vi "Draw Overlay.vi"(0 "Image (in)":T1, 1 "Image Width (in)":i32, 2 "Image Height (in)":i32, 3 "X Center (in)":sgl[](array[numeric]), 4 "Y Center (in)":sgl[](array[numeric]), 5 "Height (in)":sgl[](array[numeric]), 6 "Colors (in)":u32[](array[numeric]), 7 "Width (in)":sgl[](array[numeric]), 9 "Classes (in)":i32[](array[numeric])) -> (14 "Image (out)":T1)   [LabVIEW 2016]
uses:
  <vilib>/vision/Image Controls.llb/IMAQ Image.ctl
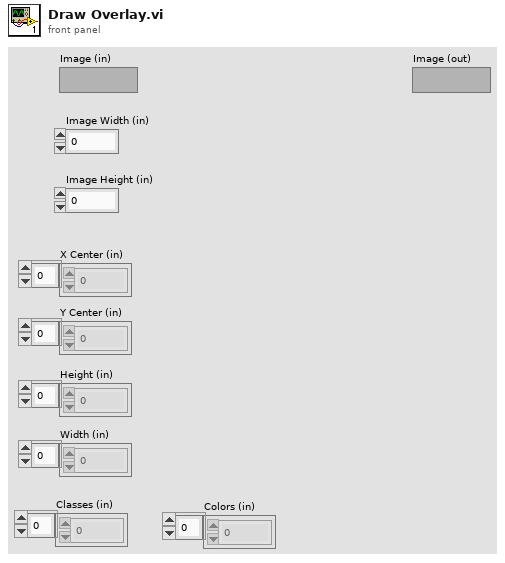
[diagram p1: front panel]
types:
  T1 = typedef "IMAQ Image.ctl" = refnum<image>
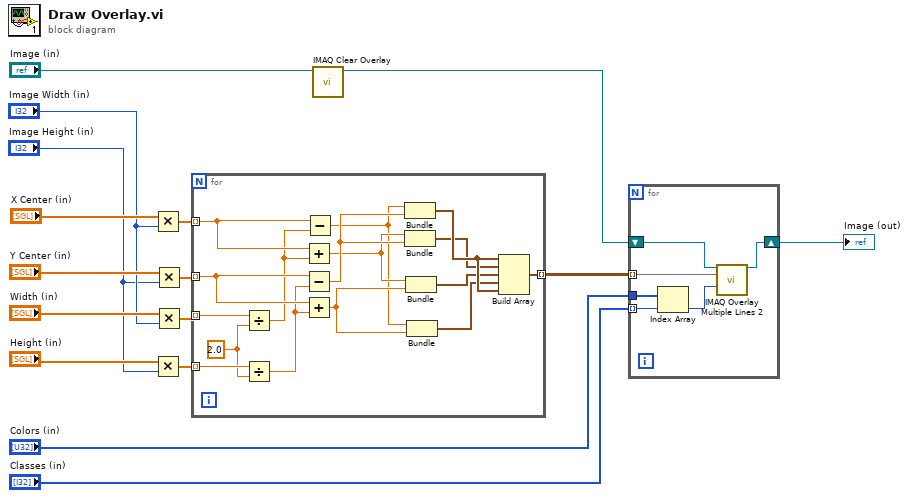
[diagram p0: block diagram]
diagram:
  n1 = Multiply(x="X Center (in)", y="Image Width (in)") -> (x*y=w4:sgl[])
  n2 = Multiply(x="Height (in)", y="Image Height (in)") -> (x*y=w7:sgl[])
  n3 = Multiply(x="Y Center (in)", y="Image Height (in)") -> (x*y=w5:sgl[])
  n4 = Multiply(x="Width (in)", y="Image Width (in)") -> (x*y=w6:sgl[])
  n5 = for {
    tunnel: w4 -> [w25] mode=indexing
    tunnel: w5 -> [w24] mode=indexing
    tunnel: w6 -> [w28] mode=indexing
    tunnel: w7 -> [w27] mode=indexing
    tunnel: [w17] -> w2 mode=indexing
    w26 = 2.0
    n6 = Divide(x=w28, y=w26) -> (x/y=w23:dbl)
    n7 = Divide(x=w27, y=w26) -> (x/y=w22:dbl)
    n8 = Add(x=w25, y=w23) -> (x+y=w20:dbl)
    n9 = Subtract(x=w24, y=w22) -> (x-y=w21:dbl)
    n10 = Add(x=w24, y=w22) -> (x+y=w19:dbl)
    n11 = Subtract(x=w25, y=w23) -> (x-y=w18:dbl)
    n12 = Bundle(w18, w21) -> (w32:cluster{dbl, dbl})  [unwired: 1 in]
    n13 = Bundle(w20, w21) -> (w29:cluster{dbl, dbl})  [unwired: 1 in]
    n14 = Bundle(w20, w19) -> (w30:cluster{dbl, dbl})  [unwired: 1 in]
    n15 = Bundle(w18, w19) -> (w31:cluster{dbl, dbl})  [unwired: 1 in]
    n16 = Build Array(w32, w29, w30, w31, w32) -> (w17:cluster{dbl, dbl}[])
  }
  n17 = call "IMAQ Clear Overlay"("Image"="Image (in)") -> ("Image Out"=w16:T1)  [unwired: 9 in, 1 out]
  n18 = for {
    tunnel: w2 -> [w38] mode=indexing
    shift-right: [w36] -> w3
    shift-left: w16 -> [w37]
    tunnel: "Classes (in)" -> [w35] mode=indexing
    tunnel: "Colors (in)" -> [w33]
    n19 = Index Array(array=w33, index=w35) -> (element=w34:u32)
    n20 = call "IMAQ Overlay Multiple Lines 2"("Image"=w37, "Line End Points"=w38, "Color"=w34) -> ("Image Out"=w36:T1)  [unwired: 11 in, 1 out]
  }
  "Image (out)" <- w3
